vi "DRC_Calibrate_thermo.vi"() -> ()   [LabVIEW 2025]
doc: "Author: Scott Hannahs <sth@magnet.fsu.edu>\n\nThis software is licensed for use under the “MIT License\"\nCopyright (c) 2025 Scott Hannahs, sth@sth@magnet.sthnet.net\n\nPermission is hereby granted, free of charge, to any person obtaining a copy of this software and associated documentation files (the \"Software\"), to deal in the Software without restriction, including without limitation the rights to use, copy, modify, merge, publish, distribute, sublicense, and/or sell copies of the Software, and to permit persons to whom the Software is furnished to do so, subject to the following conditions: The above copyright notice and this permission notice shall be included in all copies or substantial portions of the Software.\n\nTHE SOFTWARE IS PROVIDED \"AS IS\", WITHOUT WARRANTY OF ANY KIND, EXPRESS OR IMPLIED, INCLUDING BUT NOT LIMITED TO THE WARRANTIES OF MERCHANTABILITY, FITNESS FOR A PARTICULAR PURPOSE AND NONINFRINGEMENT. IN NO EVENT SHALL THE AUTHORS OR COPYRIGHT HOLDERS BE LIABLE FOR ANY CLAIM, DAMAGES OR OTHER LIABILITY, WHETHER IN AN ACTION OF CONTRACT, TORT OR OTHERWISE, ARISING FROM, OUT OF OR IN CONNECTION WITH THE SOFTWARE OR THE USE OR OTHER DEALINGS IN THE SOFTWARE."
uses:
  <vilib>/Utility/file.llb/Read From Spreadsheet File (DBL).vi
  <vilib>/Utility/file.llb/Write To Spreadsheet File (DBL).vi
panel:
  out "Waveform Graph":dbl[](graph)
  in  "WRITE TO FILE":bool
  out "Set Point (K)":dbl format="%.2f"
  in  "Wait Time (sec)":dbl format="%.2f"
  out "Sample (Ohms)":dbl format="%.2f"
  out "Sample Calibration (Ohms)":dbl format="%.2f"
  out "Control (K)":dbl format="%.2f"
  in  "GPIB address Calibrate":string
  in  "GPIB address Control":string
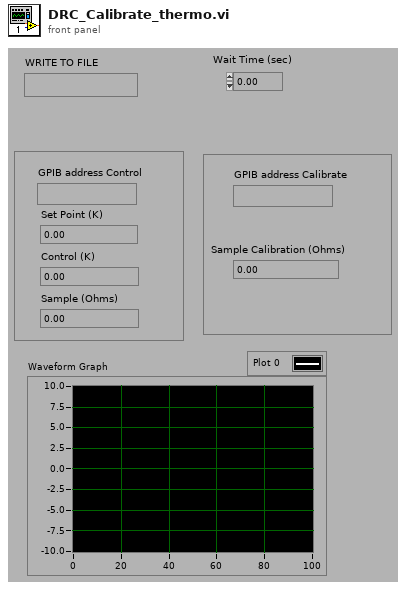
[diagram p1: front panel]
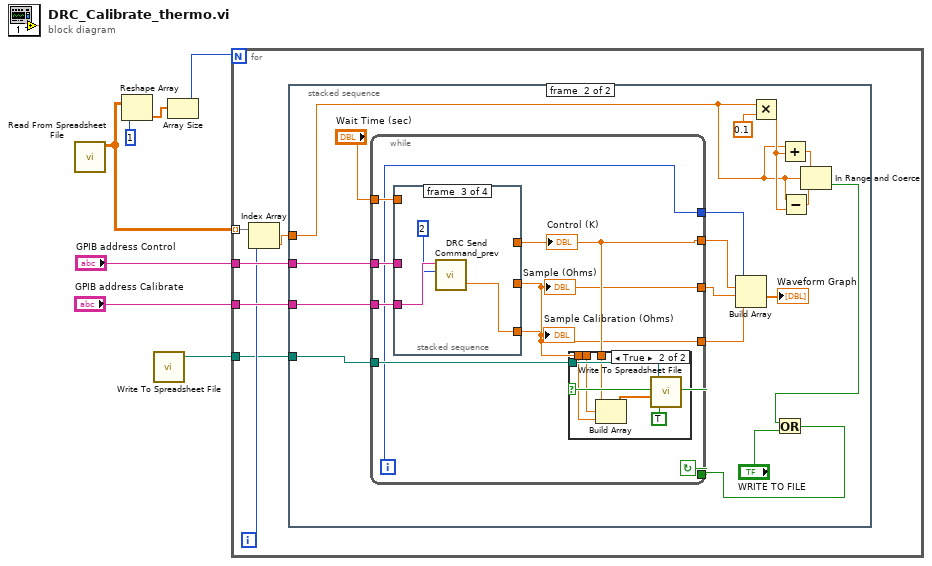
[diagram p0: block diagram]
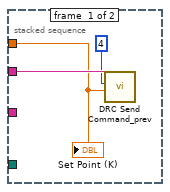
[diagram p2: hidden frame]
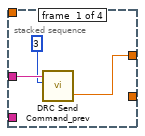
[diagram p4: hidden frame]
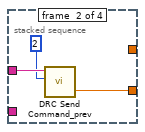
[diagram p5: hidden frame]
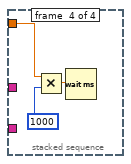
[diagram p6: hidden frame]
diagram:
  n1 = call-poly <vilib>:"Read From Spreadsheet File.vi"() -> ("all rows"=w2:dbl[][])  [unwired: 7 in, 4 out]
  n2 = Reshape Array(w2, 1) -> (w4:dbl[])
  n3 = call-poly <vilib>:"Write To Spreadsheet File.vi"() -> ("new file path (Not A Path if cancelled)"=w1:path)  [unwired: 8 in]
  n4 = Array Size(array=w4) -> (size(s)=w3:i32)
  n5 = for {
    N: w3 -> [_]
    tunnel: "GPIB address Control" -> [w13]
    tunnel: "GPIB address Calibrate" -> [w12]
    tunnel: w2 -> [w11] mode=indexing
    tunnel: w1 -> [w8]
    i -> [w10]
    n6 = Index Array(array=w11, index=w10) -> (element=w9:dbl)
    n7 = stacked-sequence {
      tunnel: w13 -> [w16 w33]
      tunnel: w12 -> [_ w32]
      tunnel: w9 -> [w15 w18]
      tunnel: w8 -> [_ w25]
      frame #0 {
        n8 = call "DRC Send Command_prev.vi"("Input"=w15, "Command"=4, "GPIB Address"=w16) -> ()  [unwired: 1 in, 2 out]
        "Set Point (K)" <- w15
      }
      frame #1 {
        n9 = Multiply(x=w18, y=0.1) -> (x*y=w20:dbl)
        n10 = Add(x=w18, y=w20) -> (x+y=w17:dbl)
        n11 = Subtract(x=w18, y=w20) -> (x-y=w19:dbl)
        n12 = In Range and Coerce(upper limit=w17, x=w18, lower limit=w19) -> (In Range?=w24:bool)  [unwired: 1 out]
        n13 = Or(x=w24, y="WRITE TO FILE") -> (x .or. y?=w22:bool)
        n14 = while {
          tunnel: [w34] -> w29
          tunnel: [w35] -> w26
          tunnel: [w36] -> w27
          tunnel: [w37] -> w28
          tunnel: "Wait Time (sec)" -> [w38]
          tunnel: w25 -> [w39]
          tunnel: w22 -> [w40]
          tunnel: w32 -> [w41]
          tunnel: w33 -> [w42]
          i -> [w34]
          stop <- w40 continue-if-true
          n15 = stacked-sequence {
            tunnel: w42 -> [w51 w54 _ _]
            tunnel: w41 -> [_ _ w57 _]
            tunnel: [_ _ w56 _] -> w35
            tunnel: [w49 _ _ _] -> w37
            tunnel: [_ w52 _ _] -> w36
            tunnel: w38 -> [_ _ _ w59]
            frame #0 {
              n16 = call "DRC Send Command_prev.vi"("Command"=3, "GPIB Address"=w51) -> ("Output"=w49:dbl)  [unwired: 2 in, 1 out]
            }
            frame #1 {
              n17 = call "DRC Send Command_prev.vi"("Command"=2, "GPIB Address"=w54) -> ("Output"=w52:dbl)  [unwired: 2 in, 1 out]
            }
            frame #2 {
              n18 = call "DRC Send Command_prev.vi"("Command"=2, "GPIB Address"=w57) -> ("Output"=w56:dbl)  [unwired: 2 in, 1 out]
            }
            frame #3 {
              n19 = Multiply(x=w59, y=1000) -> (x*y=w58:dbl)
              n20 = Wait (ms)(milliseconds to wait=w58) -> ()  [unwired: 1 out]
            }
          }
          "Control (K)" <- w37
          "Sample (Ohms)" <- w36
          "Sample Calibration (Ohms)" <- w35
          n21 = case shown="True" w40 {
            tunnel: w39 -> [_ w47]
            tunnel: w37 -> [_ w45]
            tunnel: w36 -> [_ w44]
            tunnel: w35 -> [_ w43]
            frame False {
            }
            frame True {
              n22 = Build Array(w45, w44, w43) -> (w48:dbl[])
              n23 = call-poly <vilib>:"Write To Spreadsheet File.vi"("append to file? (new file:F)"=TRUE, "1D data"=w48, "file path (dialog if empty)"=w47) -> ()  [unwired: 5 in, 1 out]
            }
          }
        }
        n24 = Build Array(w29, w28, w27, w26) -> (→"Waveform Graph":dbl[])
      }
    }
  }
